vi "Adj rf Freq for Field.vi"(6 "pts":dbl, 7 "arrayvarying":dbl[](array[numeric]), 8 "span":dbl, 11 "centfreq":dbl[](array[numeric])) -> (3 "arrayfreq":string[][](array[string]))   [LabVIEW 2009]
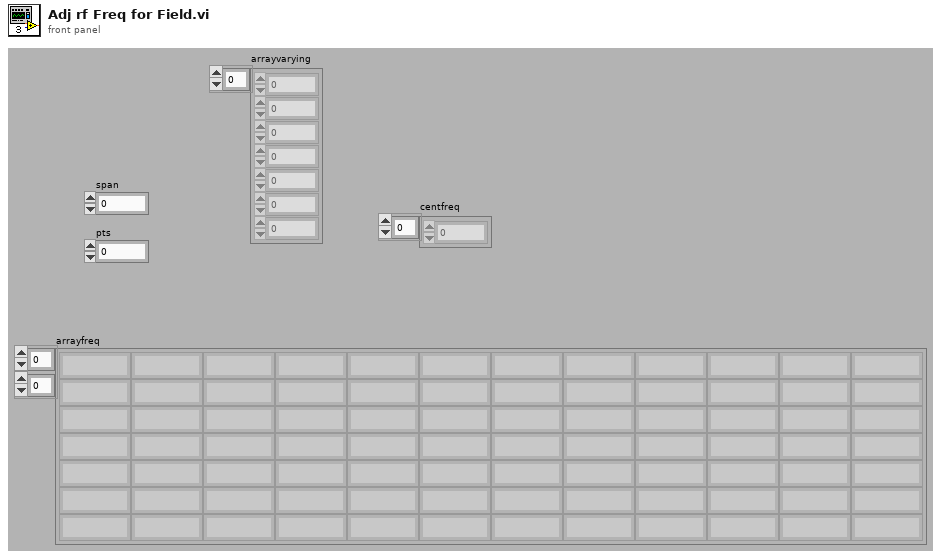
[diagram p1: front panel]
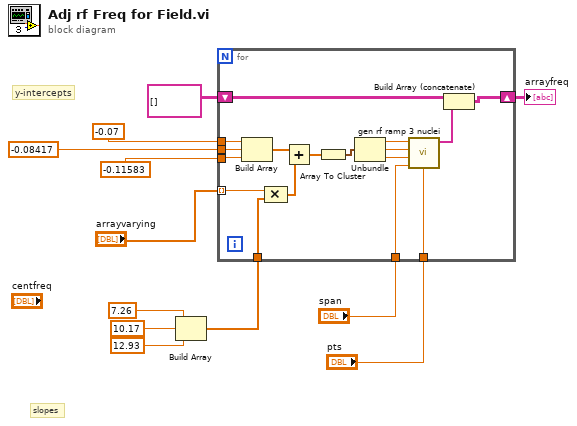
[diagram p0: block diagram]
diagram:
  # "slopes"
  # "y-intercepts"
  n1 = Build Array(7.26, 10.17, 12.93) -> (w1:dbl[])
  n2 = for {
    tunnel: -0.08417 -> [w23]
    tunnel: -0.11583 -> [w24]
    tunnel: -0.07 -> [w22]
    tunnel: "span" -> [w29]
    tunnel: "pts" -> [w28]
    shift-right: [w27] -> w9
    shift-left: string[][] [] -> [w25]
    tunnel: "arrayvarying" -> [w14] mode=indexing
    tunnel: w1 -> [w13]
    n3 = Build Array(w22, w23, w24) -> (w20:dbl[])
    n4 = Compound Arithmetic op=MULTIPLY(w14, w13) -> (w21:dbl[])
    n5 = Add(x=w20, y=w21) -> (x+y=w19:dbl[])
    n6 = Array To Cluster(array=w19) -> (cluster=w18:cluster{"[0]":dbl, "[1]":dbl, "[2]":dbl})
    n7 = Unbundle(w18) -> ("[0]"=w17:dbl, "[1]"=w16:dbl, "[2]"=w15:dbl)
    n8 = call "gen rf ramp 3 nuclei.vi"("pts"=w28, "span"=w29, "freq3"=w15, "freq2"=w16, "freq1"=w17) -> ("freqarray"=w26:string[])  [unwired: 6 out]
    n9 = Build Array (concatenate)(w25, w26) -> (w27:string[][])
  }
  "arrayfreq" <- w9
